vi "Read Allow Dropping.vi"(9 "String in":refnum<class "String.lvclass">) -> (3 "String out":refnum<class "String.lvclass">, 4 "Allow Dropping":bool)   [LabVIEW 2014, in "Raspberry Pi Compatible Compiler for LabVIEW.lvlib" / "String.lvclass"]
uses:
  String.lvclass
  String.lvclass/String.ctl
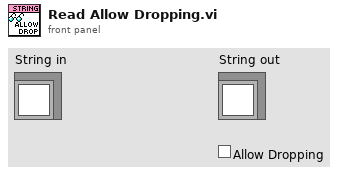
[diagram p1: front panel]
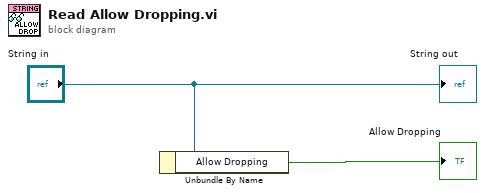
[diagram p0: block diagram]
diagram:
  n1 = Unbundle By Name("String in") -> ("Allow Dropping"=→"Allow Dropping":bool)
  "String out" <- "String in"
